vi "Drive Base Controller.vi"(8 "error in":errorcluster) -> ()   [LabVIEW 2019]
doc: "This VI executes continuously carrying out the current operation and responding to updates or new operations. It will often contain the timing or control code that is difficult to place directly in TeleOp. This VI generally opens all sensors and motors and isolates the rest of the robot code from knowing how the operations are carried out."
uses:
  <vilib>/Rock Robotics/WPI/Framework/Completion Status.ctl
  Drive Base Setpoints.ctl
  Drive Base Operations.ctl
  <vilib>/Rock Robotics/WPI/ThirdParty/REV Robotics/SPARK MAX/Typedef/Spark MAX Control Type.ctl
  <vilib>/Rock Robotics/Network Tables/NT Read Number.vi
  <vilib>/Rock Robotics/Network Tables/NT Write Boolean.vi
panel:
  in  "dimen. analysis":dbl
  in  "Interactive Values":T1
  out "Current\nCmd":string
  in  "Buttons":cluster{"Execute Cmd":bool, "Abort Cmd":bool}
  out "Command Timing":cluster{"Start Time (ms)":u32, "Iterations":i32}
  out "Status":T3
  # "Tip: It may be helpful to observe inputs and sensor values.\nYou may also want to display tuning or debugging controls."
  # "Interactive Command: You may fill in the settings for a command\nand schedule it with the Execute button. You can observe and abort\nany command while fine tuning the code for the controller."
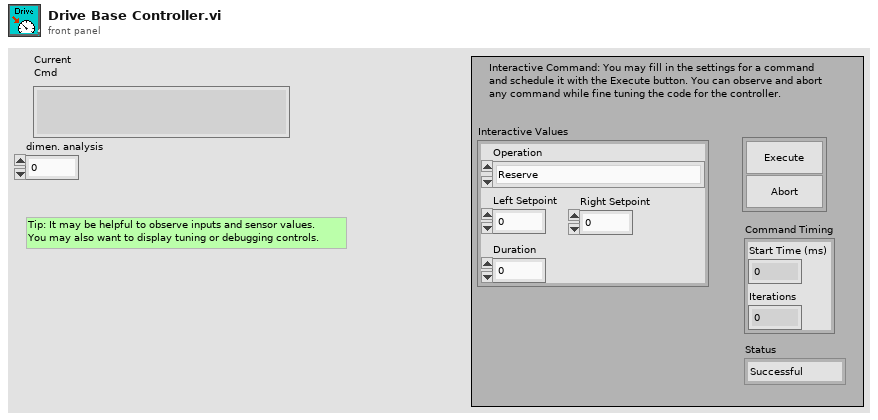
[diagram p1: front panel]
types:
  T1 = typedef "Drive Base Setpoints.ctl" = cluster{"Operation":T2, "Left Setpoint":dbl, "Duration":dbl, "Right Setpoint":dbl}
  T2 = typedef "Drive Base Operations.ctl" = enum16{"Reserve", "Read Current", "Immediate", "Limelight"}
  T3 = typedef "Completion Status.ctl" = enum16{"Successful", "Aborted", "Incomplete"}
  T4 = typedef "WPI_MotorControlDeviceRef.ctl" = cluster{"DeviceStatus":errorcluster, "Type":T5, "PWM":cluster{"PWM Channel":T6, "DeadBand":T7}, "CAN":cluster{"Device Number":u8, "SetOutput VI Ref":variant, "GetOutput VI Ref":variant, "Enable VI Ref":variant, "Disable VI Ref":variant, "Data":variant}, "Invert":bool, "DIO PWM":cluster{"PWM \"Enable\" Channel":T6, "DIOChannel":T8, "PWM Rate":dbl}}
  T5 = typedef "WPI_MotorControlType.ctl" = enum16{"PWM", "CAN", "DIO PWM"}
  T6 = typedef "FPGA_DIOPWMChannel.ctl" = enum8{"PWM 0", "PWM 1", "PWM 2", "PWM 3", "PWM 4", "PWM 5", "PWM 6", "PWM 7", "PWM 8", "PWM 9", "PWM MXP 0", "PWM MXP 1", "PWM MXP 2", "PWM MXP 3", "PWM MXP 4", "PWM MXP 5", "PWM MXP 6", "PWM MXP 7", "PWM MXP 8", "PWM MXP 9", "Invalid"}
  T7 = typedef "WPI_PWMDeadband.ctl" = cluster{"Name":string, "maxPositivePwm":i32, "minPositivePwm":i32, "centerPwm":i32, "maxNegativePwm":i32, "minNegativePwm":i32, "angularRange":u16}
  T8 = typedef "FPGA_DIOChannel.ctl" = enum8{"DIO 0", "DIO 1", "DIO 2", "DIO 3", "DIO 4", "DIO 5", "DIO 6", "DIO 7", "DIO 8", "DIO 9", "DIO MXP 0", "DIO MXP 1", "DIO MXP 2", "DIO MXP 3", "DIO MXP 4", "DIO MXP 5", "DIO MXP 6", "DIO MXP 7", "DIO MXP 8", "DIO MXP 9", "DIO MXP 10", "DIO MXP 11", "DIO MXP 12", "DIO MXP 13", "DIO MXP 14", "DIO MXP 15", "SPI Port CS1", "SPI Port CS2", "SPI Port CS3", "SPI Port MISO", "SPI Port MOSI", "Invalid"}
  T9 = typedef "Command Status Info.ctl" = cluster{"Name":string, "Status":T3, "notifier out":T10}
  T10 = typedef "Completion Notifier.ctl" = refnum<notifier>
  T11 = cluster{"Current Command":T1, "Command Timing":cluster{"Start Time (ms)":u32, "Iterations":i32}, "Command Arguments":cluster{"Command Info":T9, "Description":string, "Default Command":T1, "queue out":refnum<queue>, "Subsystem Name":string}}
  T12 = typedef "Spark MAX Control Type.ctl" = enum16{"Percent VBus", "Voltage", "Velocity", "Position", "Smart Motion", "Current", "Smart Velocity"}
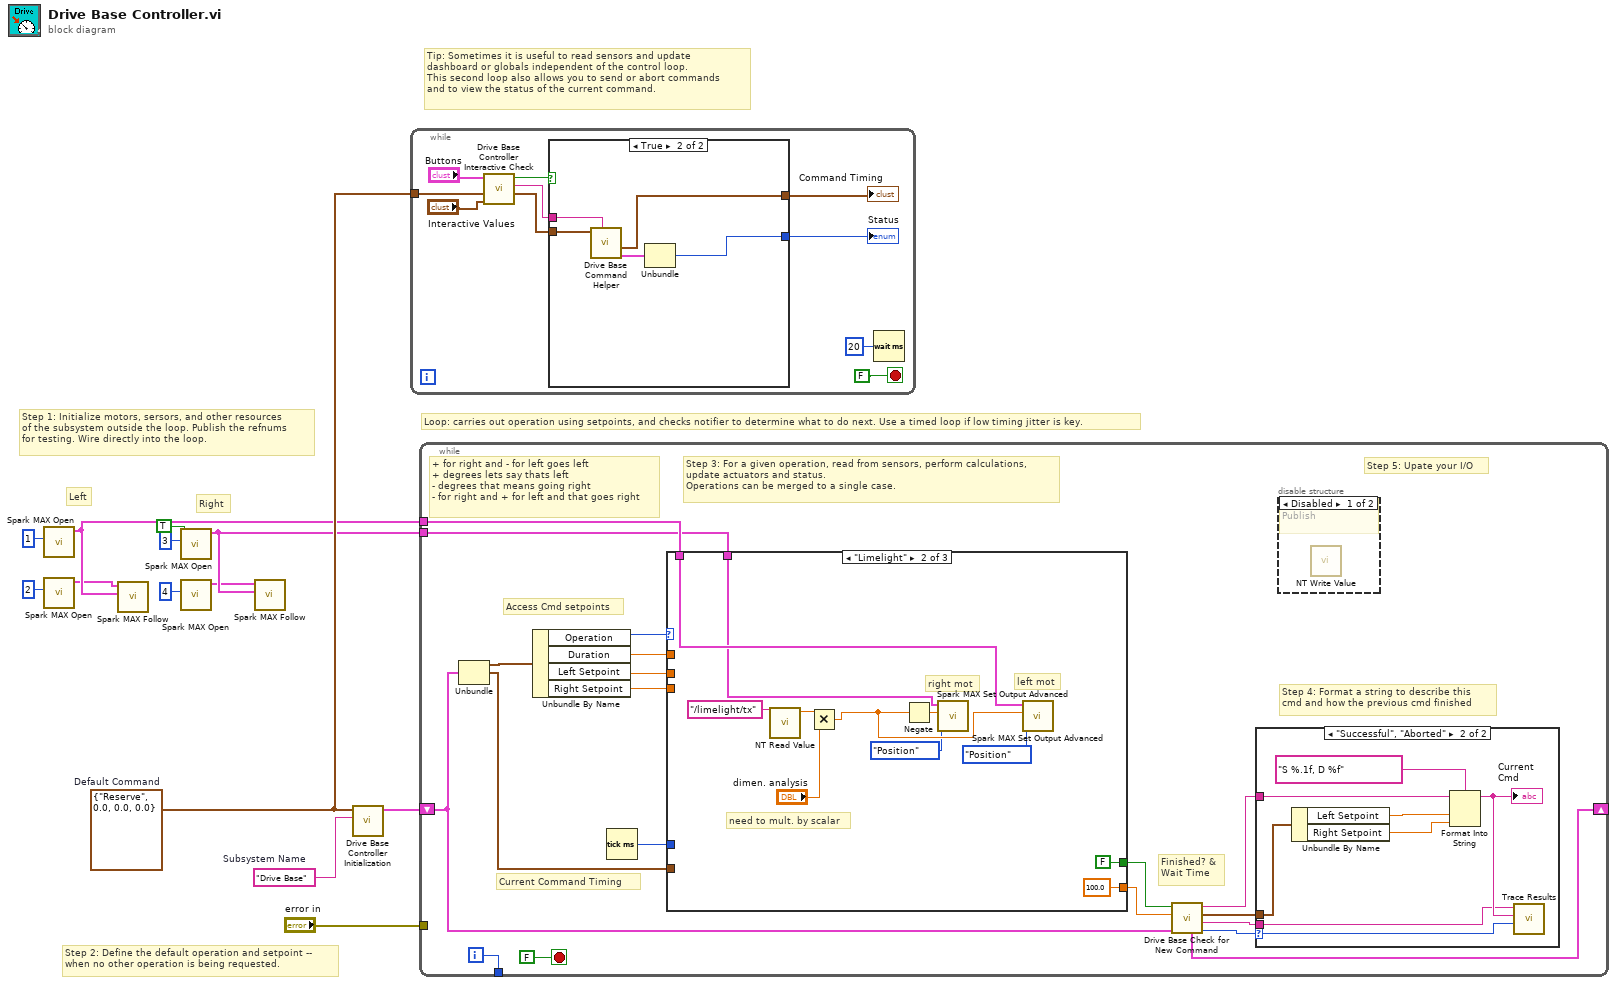
[diagram p0: block diagram]
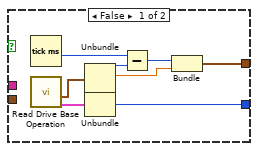
[diagram p2: hidden frame]
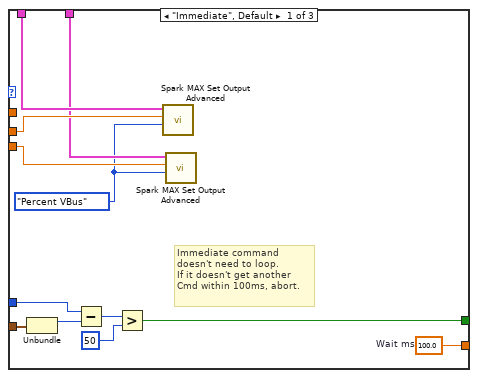
[diagram p5: hidden frame]
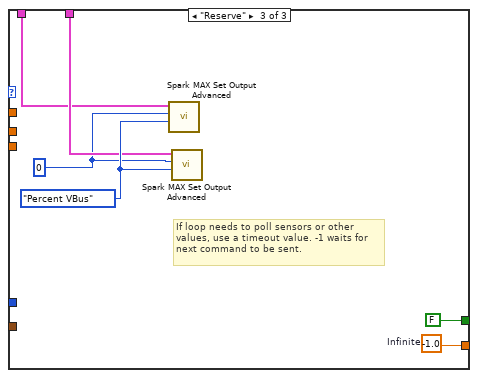
[diagram p6: hidden frame]
diagram:
  w10 = T1 {"Operation"=enum."Reserve", "Left Setpoint"=0.0, "Duration"=0.0, "Right Setpoint"=0.0}  # Default Command
  w11 = "Drive Base"  # Subsystem Name
  # "Right"
  # "Left"
  # "Tip: Sometimes it is useful to read sensors and update\ndashboard or globals independent of the control loop.\nThis second loop also allows you to send or abort commands\nand to view the status of the current command."
  # "Step 2: Define the default operation and setpoint --\nwhen no other operation is being requested."
  # "Step 1: Initialize motors, sersors, and other resources\nof the subsystem outside the loop. Publish the refnums\nfor testing. Wire directly into the loop."
  # "Loop: carries out operation using setpoints, and checks notifier to determine what to do next. Use a timed loop if low timing jitter is key."
  n1 = call <vilib>:"Spark MAX Open.vi"("Device Number"=u8 1) -> ("MotorControlDeviceRef"=w8:T4)  [unwired: 9 in, 1 out]
  n2 = call <vilib>:"Spark MAX Open.vi"("Device Number"=u8 2) -> ("MotorControlDeviceRef"=w5:T4)  [unwired: 9 in, 1 out]
  n3 = call <vilib>:"Spark MAX Follow.vi"("Master Controller"=w8, "MotorControlDeviceRef"=w5) -> ()  [unwired: 8 in, 2 out]
  n4 = call <vilib>:"Spark MAX Open.vi"("Invert"=TRUE, "Device Number"=u8 3) -> ("MotorControlDeviceRef"=w7:T4)  [unwired: 8 in, 1 out]
  n5 = call <vilib>:"Spark MAX Open.vi"("Device Number"=u8 4) -> ("MotorControlDeviceRef"=w6:T4)  [unwired: 9 in, 1 out]
  n6 = call <vilib>:"Spark MAX Follow.vi"("Master Controller"=w7, "MotorControlDeviceRef"=w6) -> ()  [unwired: 8 in, 2 out]
  n7 = call "Drive Base Controller Initialization.vi"("Subsystem Name"=w11, "Default Command"=w10) -> ("Current Command"=w12:T11)  [unwired: 9 in]
  n8 = while {
    tunnel: w10 -> [w20]
    stop <- FALSE stop-if-true
    n9 = call "Drive Base Controller Interactive Check.vi"("Interactive Command in"="Interactive Values", "Default Command"=w20, "Buttons"="Buttons") -> ("Interactive Command out"=w17:T1, "Trace String"=w18:string, "Schedule"=w19:bool)  [unwired: 6 in]
    n10 = case shown="True" w19 {
      tunnel: [w31 w36] -> w16
      tunnel: w17 -> [_ w34]
      tunnel: [w27 w32] -> w15
      tunnel: w18 -> [_ w35]
      frame False {
        n11 = Tick Count (ms)() -> (millisecond timer value=w26:u32)
        n12 = call "Read Drive Base Operation.vi"() -> ("Command Info"=w24:T9, "SubSystem Data"=w25:T1)  [unwired: 9 in, 1 out]
        n13 = Unbundle(w25) -> ("Operation"=w30:T2, "Left Setpoint"=w28:dbl)  [unwired: 2 out]
        n14 = Unbundle(w24) -> ("Status"=w31:T3)  [unwired: 2 out]
        n15 = Subtract(x=w26, y=w30) -> (x-y=w29:u32)
        n16 = Bundle(w29, "Left Setpoint"=w28) -> (w27:cluster{u32, "Left Setpoint":dbl})  [unwired: 1 in]
      }
      frame True {
        n17 = call "Drive Base Command Helper.vi"("Description"=w35, "SubSystem Data"=w34) -> ("Command Info Out"=w33:T9, "Command Timing"=w32:cluster{"Start Time (ms)":u32, "Iterations":i32})  [unwired: 7 in, 1 out]
        n18 = Unbundle(w33) -> ("Status"=w36:T3)  [unwired: 2 out]
      }
    }
    "Status" <- w16
    "Command Timing" <- w15
    n19 = Wait (ms)(milliseconds to wait=u32 20) -> ()  [unwired: 1 out]
  }
  n20 = while {
    shift-right: [w47] -> _
    shift-left: w12 -> [w40]
    tunnel: [w54] -> _
    tunnel: "error in" -> [_]
    tunnel: w8 -> [w38]
    tunnel: w7 -> [w37]
    i -> [w54]
    stop <- FALSE stop-if-true
    # "+ for right and - for left goes left\n+ degrees lets say thats left\n- degrees that means going right\n- for right and + for left and that goes right"
    # "Step 5: Upate your I/O"
    # "Step 4: Format a string to describe this\ncmd and how the previous cmd finished"
    # "Current Command Timing"
    # "Access Cmd setpoints"
    # "Finished? &\nWait Time"
    # "Step 3: For a given operation, read from sensors, perform calculations,\nupdate actuators and status.\nOperations can be merged to a single case."
    n21 = Unbundle(w40) -> ("Current Command"=w53:T1, "Command Timing"=w49:cluster{"Start Time (ms)":u32, "Iterations":i32})  [unwired: 1 out]
    n22 = Unbundle By Name(w53) -> ("Operation"=w52:T2, "Duration"=w51:dbl, "Left Setpoint"=w48:dbl, "Right Setpoint"=w39:dbl)
    n23 = Tick Count (ms)() -> (millisecond timer value=w50:u32)
    n24 = case shown="\"Limelight\"" w52 {
      tunnel: [w75 100.0 ("Infinite") w92] -> w45
      tunnel: [w69 FALSE ("ignore previous (F)") FALSE ("ignore previous (F)")] -> w46
      tunnel: w49 -> [w71 _ _]
      tunnel: w51 -> [_ _ _]
      tunnel: w50 -> [w70 _ _]
      tunnel: w48 -> [w68 _ _]
      tunnel: w39 -> [w67 _ _]
      tunnel: w38 -> [w66 w79 w88]
      tunnel: w37 -> [w65 w78 w89]
      frame "Immediate", Default {
        w64 = Spark_MAX_Control_Type."Percent VBus" ("Control Mode")
        w75 = 100.0  # Wait ms
        # "Immediate command\ndoesn't need to loop.\nIf it doesn't get another\nCmd within 100ms, abort."
        n25 = Unbundle(w71) -> ("Start Time (ms)"=w74:u32)  [unwired: 1 out]
        n26 = Subtract(x=w70, y=w74) -> (x-y=w73:u32)
        n27 = Greater?(x=w73, y=u8 50 ("Left Motor")) -> (0:w69:bool)
        n28 = call <vilib>:"Spark MAX Set Output Advanced.vi"("Control Mode"=w64, "Setpoint"=w68, "MotorControlDevRef"=w66) -> ()  [unwired: 7 in, 2 out]
        n29 = call <vilib>:"Spark MAX Set Output Advanced.vi"("Control Mode"=w64, "Setpoint"=w67, "MotorControlDevRef"=w65) -> ()  [unwired: 7 in, 2 out]
      }
      frame "Limelight" {
        # "need to mult. by scalar"
        # "left mot"
        # "right mot"
        n30 = call-poly <vilib>:"NT Read Value.vi"("Name"="/limelight/tx") -> ("Numeric"=w82:dbl)  [unwired: 9 in, 1 out]
        n31 = Multiply(x=w82, y="dimen. analysis") -> (x*y=w80:dbl)
        n32 = Negate(x=w80) -> (-x=w83:dbl)
        n33 = call <vilib>:"Spark MAX Set Output Advanced.vi"("Control Mode"=Spark_MAX_Control_Type."Position", "Setpoint"=w83, "MotorControlDevRef"=w78) -> ()  [unwired: 7 in, 2 out]
        n34 = call <vilib>:"Spark MAX Set Output Advanced.vi"("Control Mode"=Spark_MAX_Control_Type."Position", "Setpoint"=w80, "MotorControlDevRef"=w79) -> ()  [unwired: 7 in, 2 out]
      }
      frame "Reserve" {
        w87 = 0
        w90 = Spark_MAX_Control_Type."Percent VBus" ("Control Mode")
        w92 = -1.0  # Infinite
        # "If loop needs to poll sensors or other\nvalues, use a timeout value. -1 waits for\nnext command to be sent."
        n35 = call <vilib>:"Spark MAX Set Output Advanced.vi"("Control Mode"=w90, "Setpoint"=w87, "MotorControlDevRef"=w88) -> ()  [unwired: 7 in, 2 out]
        n36 = call <vilib>:"Spark MAX Set Output Advanced.vi"("Control Mode"=w90, "Setpoint"=w87, "MotorControlDevRef"=w89) -> ()  [unwired: 7 in, 2 out]
      }
    }
    n37 = call "Drive Base Check for New Command.vi"("Current Command"=w40, "Wait time (ms)"=w45, "Finished?"=w46) -> ("Completion"=w41:T3, "Subsystem Name"=w42:string, "Current Command"=w43:T1, "Initial Trace String"=w44:string, "NextCommand"=w47:T11)  [unwired: 4 in]
    n38 = case shown="\"Successful\", \"Aborted\"" w41 {
      selector: w41 -> [_ w63]
      tunnel: w44 -> [_ w59]
      tunnel: w43 -> [_ w60]
      tunnel: w42 -> [_ w56]
      frame "Incomplete", Default {
        # "Continuing current command"
      }
      frame "Successful", "Aborted" {
        # "Report and setup for next command"
        n39 = Unbundle By Name(w60) -> ("Left Setpoint"=w62:dbl, "Right Setpoint"=w57:dbl)
        n40 = Format Into String(format string="S %.1f, D %f", initial string=w59, w62, w57) -> (resulting string=w58:string)  [unwired: 1 in, 1 out]
        "Current\nCmd" <- w58
        n41 = call <vilib>:"Trace Results.vi"("Status of previous command"=w63, "Description"=w58, "Subsystem"=w56) -> ()  [unwired: 9 in]
      }
    }
    n42 = disable-structure shown="Disabled" {
      frame Disabled {
        # "Publish"
        n43 = call-poly <vilib>:"NT Write Value.vi"() -> ()  [unwired: 11 in, 1 out]
      }
      frame Enabled {
      }
    }
  }
